vi "set channel.vi"(8 "error in":errorcluster, 10 "Modbus Module Channel.lvclass":refnum<class "Modbus Module Channel.lvclass">, 11 "Modbus Slave configuration in":refnum<class "Modbus Slave configuration.lvclass">) -> (0 "error out":errorcluster, 3 "Modbus Slave configuration out":refnum<class "Modbus Slave configuration.lvclass">)   [LabVIEW 2013, in "Modbus Slave configuration.lvclass"]
doc: "This function is responsible for replacing a channel, by name in the configuration class.Platypus Framework 1.0.1.65\nNI Systems Engineering - National Instruments"
uses:
  Modbus Slave configuration.lvclass
  module channel/Modbus Module Channel.lvclass
  <vilib>/NI/Tag Bus/tag/tag descriptor.lvclass/tag descriptor.ctl
  Modbus Slave configuration.lvclass/Modbus Slave configuration.ctl
  <vilib>/NI/Tag Bus/tag/tag descriptor.lvclass
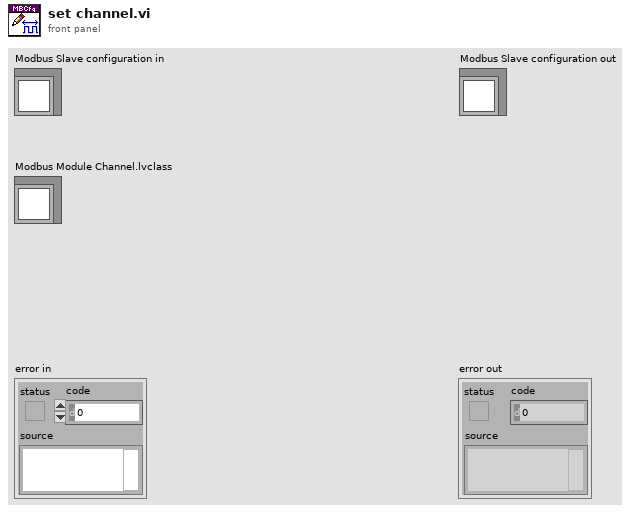
[diagram p1: front panel]
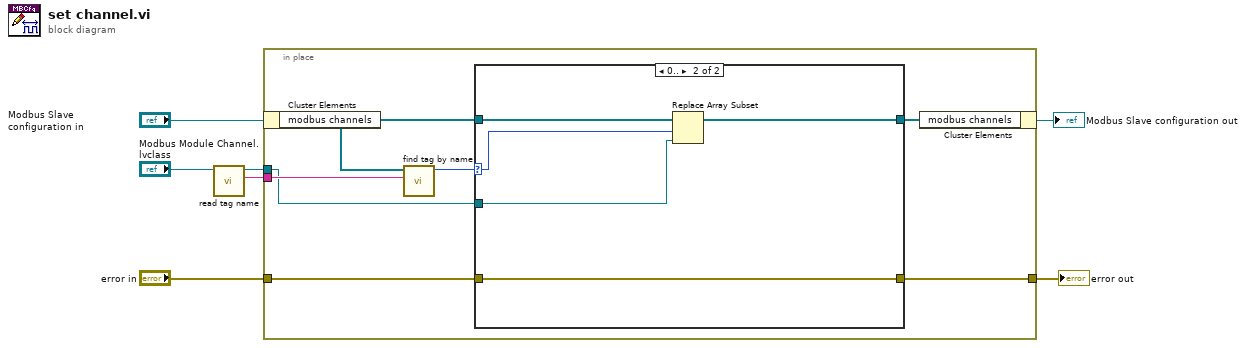
[diagram p0: block diagram]
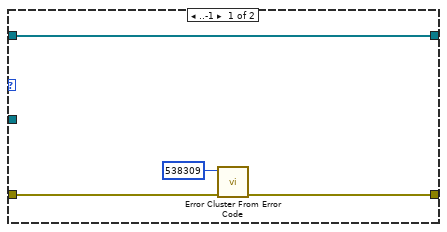
[diagram p2: hidden frame]
diagram:
  n1 = call <vilib>:"read tag name.vi"("system tag in"="Modbus Module Channel.lvclass") -> ("name"=w6:string, "system tag out"=w7:refnum<class "Modbus Module Channel.lvclass">)  [unwired: 8 in, 1 out]
  n2 = in-place {
    in-place-border: [w13] -> w4
    in-place-border: "error in" -> [w11]
    in-place-border: w7 -> [w9]
    in-place-border: w6 -> [w10]
    n3 = in-place-cluster #1("Modbus Slave configuration in") -> ("modbus channels"=w14:refnum<class "Modbus Module Channel.lvclass">[])
    n4 = call <vilib>:"find tag by name.vi"("name"=w10, "tags in"=w14) -> ("index"=w8:i32)  [unwired: 9 in]
    n5 = case shown="0.." w8 {
      selector: w8 -> [_ w19]
      tunnel: w14 -> [w16 w22]
      tunnel: [w17 w23] -> w13
      tunnel: [w16 w21] -> w12
      tunnel: w11 -> [w15 w23]
      tunnel: w9 -> [_ w20]
      frame ..-1 {
        n6 = call <vilib>:"Error Cluster From Error Code.vi"("error in (no error)"=w15, "error code (0)"=538309) -> ("error out"=w17:errorcluster)  [unwired: 7 in]
      }
      frame 0.. {
        n7 = Replace Array Subset(array=w22, new element=w20, index=w19) -> (w21:refnum<class "Modbus Module Channel.lvclass">[])
      }
    }
    n8 = in-place-cluster #1("modbus channels"=w12) -> (→"Modbus Slave configuration out":refnum<class "Modbus Slave configuration.lvclass">)
  }
  "error out" <- w4
